vi "GetScans.vi"(7 "condition":string, 8 "error in (no error)":errorcluster, 9 "exp_date":string, 10 "mouse_id":dbl, 11 "Database in":refnum<class "Database.lvclass">) -> (0 "error out":errorcluster, 2 "Scan Clusters":T1(array[cluster]), 3 "Database out":refnum<class "Database.lvclass">)   [LabVIEW 2011, in "Database.lvclass"]
uses:
  Database.lvclass
  Database.lvclass/Database.ctl
  <vilib>/addons/database/_DB Variant To Data/Database Variant To Data.xnode
  <vilib>/addons/database/NI_Database_API.lvlib
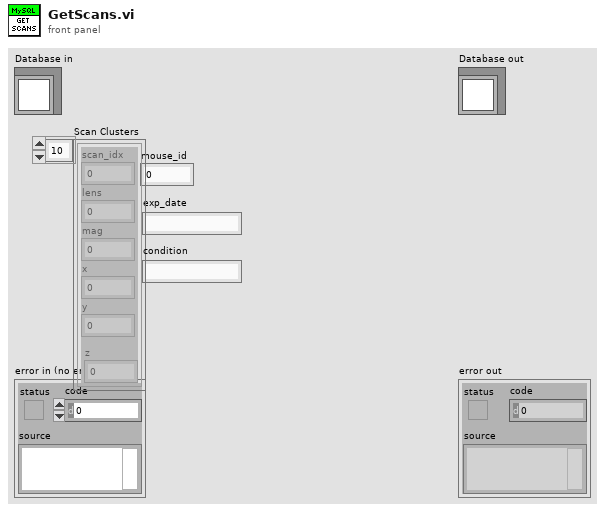
[diagram p1: front panel]
types:
  T1 = cluster{"scan_idx":dbl, "lens":dbl, "mag":dbl, "x":dbl, "y":dbl, "z":dbl}[]
  T2 = typedef "NI_Database_API.lvlib/Conn ObjectReference.ctl" = refnum<k1>
  T3 = cluster{"data[0]":dbl, "data[1]":dbl, "data[2]":dbl, "data[3]":dbl, "data[4]":dbl, "data[5]":dbl}
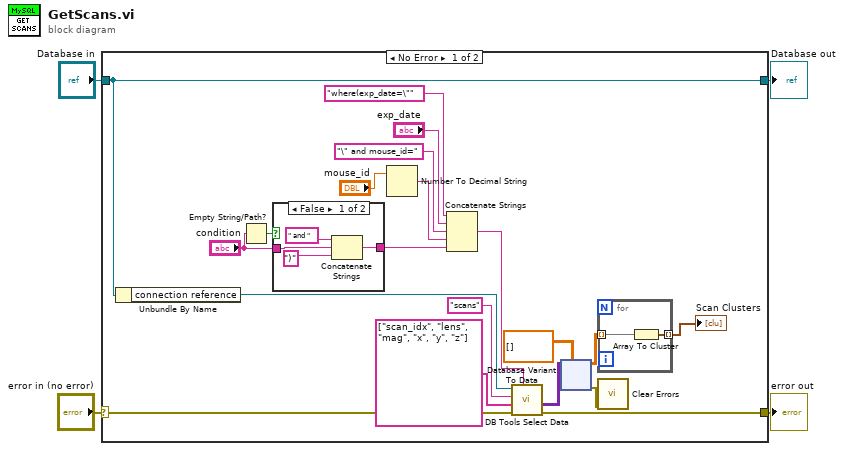
[diagram p0: block diagram]
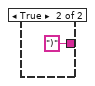
[diagram p2: hidden frame]
diagram:
  n1 = case shown="No Error" "error in (no error)" {
    selector: "error in (no error)" -> [w22 w77]
    tunnel: [w7 w77] -> w3
    tunnel: [w13 w76] -> w1
    tunnel: "Database in" -> [w13 w76]
    frame No Error {
      n2 = Unbundle By Name(w13) -> ("connection reference"=w24:T2)
      n3 = Empty String/Path?(string/path="condition") -> (empty?=w9:bool)
      n4 = case shown="False" w9 {
        tunnel: [w25 ")"] -> w10
        tunnel: "condition" -> [w27 _]
        frame False {
          n5 = Concatenate Strings(" and " ("string"), w27, ")" ("string")) -> (w25:string)
        }
        frame True {
        }
      }
      n6 = Number To Decimal String(number="mouse_id") -> (decimal integer string=w17:string)  [unwired: 1 in]
      n7 = Concatenate Strings("where(exp_date=\"", "exp_date", "\" and mouse_id=", w17, w10) -> (w15:string)
      n8 = call <vilib>:"DB Tools Select Data.vi"("condition"=w15, "error in (no error)"=w22, "columns"=string[] ["scan_idx", "lens", "mag", "x", "y", "z"], "table"="scans", "connection reference"=w24) -> ("error out"=w7:errorcluster, "data"=w11:variant[][])  [unwired: 1 in, 1 out]
      n9 = xnode "Database Variant To Data"("database variant"=w11, "type"=dbl[][] []) -> ("data"=w12:dbl[][], "error out"=w6:errorcluster)  [unwired: 1 in]
      n10 = for {
        tunnel: w12 -> [w31] mode=indexing
        tunnel: [w30] -> w5 mode=indexing
        n11 = Array To Cluster(array=w31) -> (cluster=w30:T3)
      }
      "Scan Clusters" <- w5
      n12 = call <vilib>:"Clear Errors.vi"("error in (no error)"=w6) -> ()  [unwired: 6 in, 1 out]
    }
    frame Error {
    }
  }
  "error out" <- w3
  "Database out" <- w1
